vi "CRYWindows Correction.vi"(2 "window":T1 items=["Rectangle"=0, "Hanning"=1, "Hamming"=2, "Blackman-Harris"=3, "Exact Blackman"=4, "Blackman"=5, "Flat Top"=6, "4 Term B-Harris "=7, "7 Term B-Harris"=8, "Low Sidelobe"=9, "Blackman Nuttall"=11, "Triangle"=30, "Bartlett-Hanning"=31, "Bohman"=32, "Parzen"=33, "Welch"=34, "Kaiser"=60, "Dolph-Chebyshev"=61, "Gaussian"=62], 4 "N Sine":i32, 5 "N FFT":i32, 6 "Frequnecy":dbl, 7 "Sampling rate":dbl) -> (0 "Index":i16, 1 "Complex Correction":cdb)   [LabVIEW 2013]
uses:
  <vilib>/Analysis/4window.llb/windowTd.ctl
  <vilib>/Analysis/2dsp.llb/Real FFT.vi
  <vilib>/Analysis/0measdsp.llb/Scaled Time Domain Window (DBL).vi
  <vilib>/Analysis/2dsp.llb/Zero Padder (DBL).vi
  <vilib>/measure/NI_MABase.lvlib
  <vilib>/Analysis/NI_AALPro.lvlib
panel:
  out "error out":errorcluster
  in  "error in (no error)":errorcluster
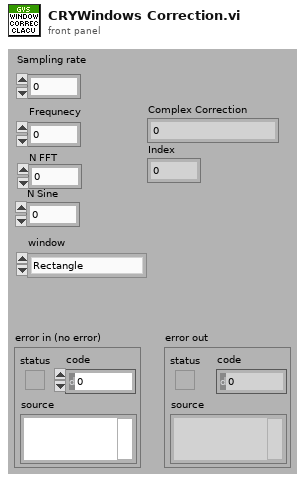
[diagram p1: front panel]
types:
  T1 = typedef "NI_AALPro.lvlib/windowTd.ctl" = u32
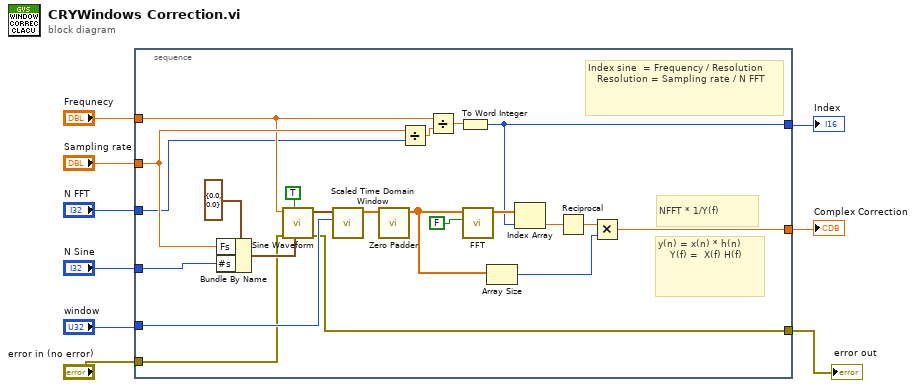
[diagram p0: block diagram]
diagram:
  n1 = stacked-sequence {
    tunnel: "Sampling rate" -> [w21]
    tunnel: "N FFT" -> [w12]
    tunnel: "Frequnecy" -> [w17]
    tunnel: [w24] -> w5
    tunnel: [w29] -> w4
    tunnel: "N Sine" -> [w27]
    tunnel: "window" -> [w20]
    tunnel: "error in (no error)" -> [w11]
    tunnel: [w10] -> w1
    frame #0 {
      # "NFFT * 1/Y(f)"
      # "y(n) = x(n) * h(n) \n    Y(f) =  X(f) H(f)"
      # "Index sine  = Frequency / Resolution\n   Resolution = Sampling rate / N FFT"
      n2 = Bundle By Name(cluster=cluster{"Fs":dbl, "#s":dbl} {"Fs"=0.0, "#s"=0.0} ("sampling info"), "Fs"=w21, "#s"=w27) -> (w13:cluster{"Fs":dbl, "#s":dbl})
      n3 = call <vilib>:"Sine Waveform.vi"("sampling info"=w13, "reset signal"=TRUE, "error in (no error)"=w11, "frequency"=w17) -> ("error out"=w10:errorcluster, "signal out"=w18:waveform(dbl))  [unwired: 3 in, 3 out]
      n4 = call-poly <vilib>:"Scaled Time Domain Window.vi"("window"=w20, "X"=w18) -> ("Windowed X"=w16:dbl[])  [unwired: 1 in, 8 out]
      n5 = call-poly <vilib>:"Zero Padder.vi"("Input Array"=w16) -> ("Zero Padded Array"=w25:dbl[])  [unwired: 1 in, 9 out]
      n6 = Divide(x=w21, y=w12) -> (x/y=w31:dbl)
      n7 = Divide(x=w17, y=w31) -> (x/y=w30:dbl)
      n8 = To Word Integer(number=w30) -> (16bit integer=w24:i16)
      n9 = call-poly <vilib>:"FFT.vi"("shift?"=FALSE, "X"=w25) -> ("FFT {X}"=w26:cdb[])  [unwired: 1 in, 8 out]
      n10 = Array Size(array=w25) -> (size(s)=w15:i32)
      n11 = Index Array(array=w26, index=w24) -> (element=w23:cdb)
      n12 = Reciprocal(x=w23) -> (1/x=w19:cdb)
      n13 = Multiply(x=w19, y=w15) -> (x*y=w29:cdb)
    }
  }
  "Complex Correction" <- w4
  "Index" <- w5
  "error out" <- w1
